vi "add_uint64.vi"   [LabVIEW 2015]
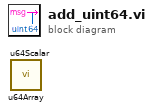
[diagram p0: block diagram]
diagram:
  n1 = call "u64Array.vi"() -> ()  [unwired: 5 in, 1 out]
  n2 = call "u64Scalar.vi"() -> ()  [unwired: 5 in, 1 out]
